vi "Test TEC.vi"() -> ()   [LabVIEW 2014, in "TE Cooler.lvlib"]
uses:
  TE Cooler.lvlib
  TE Cooler.lvclass
  Data/TECData.lvclass
  Controls/Sensor Type.ctl
  Controls/Units.ctl
panel:
  out "T1":sgl
  out "T2":sgl
  out "error out 2":errorcluster
  out "error out":errorcluster={"status"=TRUE, "code"=-1073807339, "source"="VISA Read in Serial IO.lvclass:Cmd to R_W - Synchronous.vi->TE Cooler.lvlib:TE Cooler.lvclass:Write to Port.vi->TE Cooler.lvlib:TE Cooler.lvclass:Init.vi->cPAS.lvclass:Serial Config.vi->cPAS.lvclass:Start Config.vi->PAS.lvclass:Configure.vi->PAS Server.vi->Combined Server.vi"}
  out "Power":dbl
  out "T":dbl
  in  "SP":sgl
  out "units":T1
  out "DataOut":dbl
  out "sense_type":T2
  in  "stop":bool
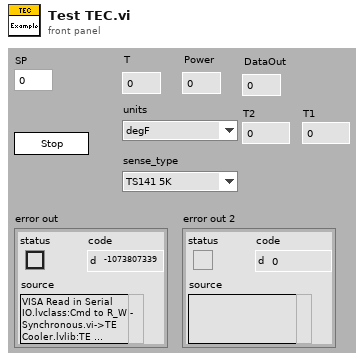
[diagram p1: front panel]
types:
  T1 = typedef "TE Cooler.lvlib/TE Cooler.lvclass/Units.ctl" = enum16{"degF", "degC"}
  T2 = typedef "TE Cooler.lvlib/TE Cooler.lvclass/Sensor Type.ctl" = enum16{"TS141 5K", "TS67 OR TS136 15K", "TS91 10K", "TS165 230K", "TS104 50K", "YSI H TP53 10K"}
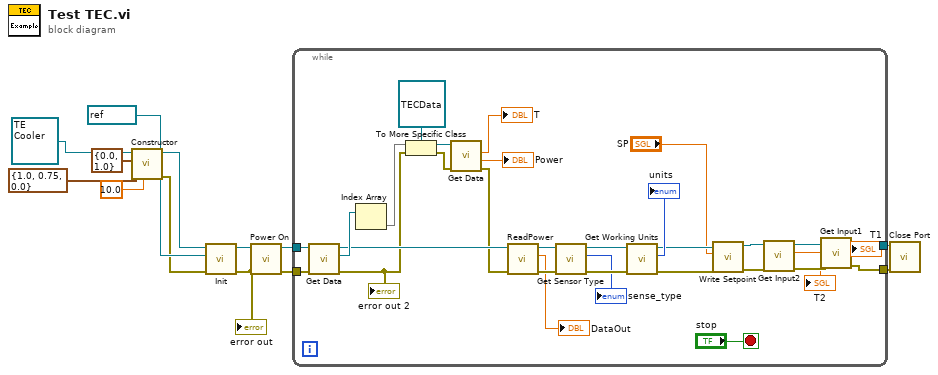
[diagram p0: block diagram]
diagram:
  n1 = call "Constructor.vi"("TSP"=sgl 10.0, "PID Params"=cluster{"P":sgl, "I":sgl, "D":sgl} {"P"=1.0, "I"=0.75, "D"=0.0}, "Ctl Params"=cluster{"htx":sgl, "clx":sgl} {"htx"=0.0, "clx"=1.0}, "TE Cooler in"=refnum<class "TE Cooler.lvclass"> refnum ("TE Cooler.lvclass")) -> ("error out"=w1:errorcluster, "TE Cooler out"=w2:refnum<class "TE Cooler.lvclass">)  [unwired: 6 in]
  n2 = call-dynamic "Init.vi"("error in"=w1, 10:refnum<visa-resource-name> "TEC" ("Port"), "TE Cooler in"=w2) -> ("error out"=w9:errorcluster, "TE Cooler out"=w10:refnum<class "TE Cooler.lvclass">)  [unwired: 6 in, 1 out]
  "error out" <- w9
  n3 = call "Power On.vi"("error in"=w9, "TE Cooler in"=w10) -> ("error out"=w7:errorcluster, "TE Cooler out"=w8:refnum<class "TE Cooler.lvclass">)  [unwired: 8 in]
  n4 = while {
    tunnel: w8 -> [w33]
    tunnel: w7 -> [w32]
    tunnel: [w19] -> w12
    tunnel: [w18] -> w11
    stop <- "stop" stop-if-true
    n5 = call-dynamic "Get Data.vi"("error in"=w32, "TE Cooler in"=w33) -> ("error out"=w24:errorcluster, "Data Out"=w29:refnum<class "Data.lvclass">, "TE Cooler out"=w25:refnum<class "TE Cooler.lvclass">)  [unwired: 7 in]
    "error out 2" <- w24
    n6 = Index Array(array=w29) -> (element=w28)  [unwired: 1 in]
    n7 = To More Specific Class(target class=refnum<class "TECData.lvclass"> refnum ("TECData.lvclass"), reference=w28, error in=w24) -> (specific class reference=w30:refnum<class "TECData.lvclass">, error out=w23:errorcluster)
    n8 = call "Get Data.vi"("error in (no error)"=w23, "TECData in"=w30) -> ("error out"=w22:errorcluster, "Power"=→"Power":sgl, "T"=→"T":sgl)  [unwired: 6 in, 1 out]
    n9 = call "ReadPower.vi"("error in"=w22, "TE Cooler in"=w25) -> ("error out"=w42:errorcluster, "Power (%)"=→"DataOut":sgl, "TE Cooler out"=w43:refnum<class "TE Cooler.lvclass">)  [unwired: 7 in]
    n10 = call "Get Sensor Type.vi"("error in"=w42, "TE Cooler in"=w43) -> ("error out"=w40:errorcluster, "sense_type"=→"sense_type":T2, "TE Cooler out"=w41:refnum<class "TE Cooler.lvclass">)  [unwired: 7 in]
    n11 = call "Get Working Units.vi"("error in"=w40, "TE Cooler in"=w41) -> ("error out"=w36:errorcluster, "units"=→"units":T1, "TE Cooler out"=w35:refnum<class "TE Cooler.lvclass">)  [unwired: 7 in]
    n12 = call "Write Setpoint.vi"("error in"=w36, "SP"="SP", "TE Cooler in"=w35) -> ("error out"=w16:errorcluster, "TE Cooler out"=w21:refnum<class "TE Cooler.lvclass">)  [unwired: 7 in]
    n13 = call "Get Input2.vi"("error in"=w16, "TE Cooler in"=w21) -> ("error out"=w17:errorcluster, "T2"=→"T2":sgl, "TE Cooler out"=w20:refnum<class "TE Cooler.lvclass">)  [unwired: 7 in]
    n14 = call "Get Input1.vi"("error in"=w17, "TE Cooler in"=w20) -> ("error out"=w18:errorcluster, "T1"=→"T1":sgl, "TE Cooler out"=w19:refnum<class "TE Cooler.lvclass">)  [unwired: 7 in]
  }
  n15 = call-dynamic "Close Port.vi"("error in (no error)"=w11, "Serial IO in"=w12) -> ()  [unwired: 8 in, 2 out]
